vi "Make Defect Pair.vi"(4 "Maximum Distnce":dbl=12.0, 6 "Minimum Distance":dbl=11.0, 8 "Defect 2":cluster{"Species":string, "Defect Type":string}={"Species"="Te", "Defect Type"="Interstitial, Tetra, Unlike atoms"}, 9 "Defect 1":cluster{"Species":string, "Defect Type":string}={"Species"="Te", "Defect Type"="Substitutional"}, 10 "Defect 1 Atom Index":i32=10, 11 "Input Structure":T1={"Structure Name"="Gamma8_64atom", "Lattice vector a"=[13.21796569573, 0.0, 0.0], "Lattice vector b"=[0.0, 13.21796569573, 0.0], "Lattice vector c"=[0.0, 0.0, 13.21796569573], "Atoms Array"=[{"Atom Name"="Cd", "Positions (Direct)"=[[0.0, 0.0, 0.0], [0.0, 0.0, 0.5], [0.0, 0.5, 0.0], [0.0, 0.5, 0.5], [0.5, 0.0, 0.0], [0.5, 0.0, 0.5], [0.5, 0.5, 0.0], [0.5, 0.5, 0.5], [0.0, 0.25, 0.25], [0.0, 0.25, 0.75], [0.0, 0.75, 0.25], [0.0, 0.75, 0.75], [0.5, 0.25, 0.25], [0.5, 0.25, 0.75], [0.5, 0.75, 0.25], [0.5, 0.75, 0.75], [0.25, 0.0, 0.25], [0.25, 0.0, 0.75], [0.25, 0.5, 0.25], [0.25, 0.5, 0.75], [0.75, 0.0, 0.25], [0.75, 0.0, 0.75], [0.75, 0.5, 0.25], [0.75, 0.5, 0.75], [0.25, 0.25, 0.0], [0.25, 0.25, 0.5], [0.25, 0.75, 0.0], [0.25, 0.75, 0.5], [0.75, 0.25, 0.0], [0.75, 0.25, 0.5], [0.75, 0.75, 0.0], [0.75, 0.75, 0.5]], "Positions (Cartesian)"=[[0.0, 0.0, 0.0], [0.0, 0.0, 6.608982847865], [0.0, 6.608982847865, 0.0], [0.0, 6.608982847865, 6.608982847865], [6.608982847865, 0.0, 0.0], [6.608982847865, 0.0, 6.608982847865], [6.608982847865, 6.608982847865, 0.0], [6.608982847865, 6.608982847865, 6.608982847865], [0.0, 3.3044914239325, 3.3044914239325], [0.0, 3.3044914239325, 9.913474271797499], [0.0, 9.913474271797499, 3.3044914239325], [0.0, 9.913474271797499, 9.913474271797499], [6.608982847865, 3.3044914239325, 3.3044914239325], [6.608982847865, 3.3044914239325, 9.913474271797499], [6.608982847865, 9.913474271797499, 3.3044914239325], [6.608982847865, 9.913474271797499, 9.913474271797499], [3.3044914239325, 0.0, 3.3044914239325], [3.3044914239325, 0.0, 9.913474271797499], [3.3044914239325, 6.608982847865, 3.3044914239325], [3.3044914239325, 6.608982847865, 9.913474271797499], [9.913474271797499, 0.0, 3.3044914239325], [9.913474271797499, 0.0, 9.913474271797499], [9.913474271797499, 6.608982847865, 3.3044914239325], [9.913474271797499, 6.608982847865, 9.913474271797499], [3.3044914239325, 3.3044914239325, 0.0], [3.3044914239325, 3.3044914239325, 6.608982847865], [3.3044914239325, 9.913474271797499, 0.0], [3.3044914239325, 9.913474271797499, 6.608982847865], [9.913474271797499, 3.3044914239325, 0.0], [9.913474271797499, 3.3044914239325, 6.608982847865], [9.913474271797499, 9.913474271797499, 0.0], [9.913474271797499, 9.913474271797499, 6.608982847865]]}, {"Atom Name"="Te", "Positions (Direct)"=[[0.125, 0.125, 0.125], [0.125, 0.125, 0.625], [0.125, 0.625, 0.125], [0.125, 0.625, 0.625], [0.625, 0.125, 0.125], [0.625, 0.125, 0.625], [0.625, 0.625, 0.125], [0.625, 0.625, 0.625], [0.375, 0.375, 0.125], [0.375, 0.375, 0.625], [0.375, 0.875, 0.125], [0.375, 0.875, 0.625], [0.875, 0.375, 0.125], [0.875, 0.375, 0.625], [0.875, 0.875, 0.125], [0.875, 0.875, 0.625], [0.375, 0.125, 0.375], [0.375, 0.125, 0.875], [0.375, 0.625, 0.375], [0.375, 0.625, 0.875], [0.875, 0.125, 0.375], [0.875, 0.125, 0.875], [0.875, 0.625, 0.375], [0.875, 0.625, 0.875], [0.125, 0.375, 0.375], [0.125, 0.375, 0.875], [0.125, 0.875, 0.375], [0.125, 0.875, 0.875], [0.625, 0.375, 0.375], [0.625, 0.375, 0.875], [0.625, 0.875, 0.375], [0.625, 0.875, 0.875]], "Positions (Cartesian)"=[[1.65224571196625, 1.65224571196625, 1.65224571196625], [1.65224571196625, 1.65224571196625, 8.261228559831249], [1.65224571196625, 8.261228559831249, 1.65224571196625], [1.65224571196625, 8.261228559831249, 8.261228559831249], [8.261228559831249, 1.65224571196625, 1.65224571196625], [8.261228559831249, 1.65224571196625, 8.261228559831249], [8.261228559831249, 8.261228559831249, 1.65224571196625], [8.261228559831249, 8.261228559831249, 8.261228559831249], [4.9567371358987495, 4.9567371358987495, 1.65224571196625], [4.9567371358987495, 4.9567371358987495, 8.261228559831249], [4.9567371358987495, 11.56571998376375, 1.65224571196625], [4.9567371358987495, 11.56571998376375, 8.261228559831249], [11.56571998376375, 4.9567371358987495, 1.65224571196625], [11.56571998376375, 4.9567371358987495, 8.261228559831249], [11.56571998376375, 11.56571998376375, 1.65224571196625], [11.56571998376375, 11.56571998376375, 8.261228559831249], [4.9567371358987495, 1.65224571196625, 4.9567371358987495], [4.9567371358987495, 1.65224571196625, 11.56571998376375], [4.9567371358987495, 8.261228559831249, 4.9567371358987495], [4.9567371358987495, 8.261228559831249, 11.56571998376375], [11.56571998376375, 1.65224571196625, 4.9567371358987495], [11.56571998376375, 1.65224571196625, 11.56571998376375], [11.56571998376375, 8.261228559831249, 4.9567371358987495], [11.56571998376375, 8.261228559831249, 11.56571998376375], [1.65224571196625, 4.9567371358987495, 4.9567371358987495], [1.65224571196625, 4.9567371358987495, 11.56571998376375], [1.65224571196625, 11.56571998376375, 4.9567371358987495], [1.65224571196625, 11.56571998376375, 11.56571998376375], [8.261228559831249, 4.9567371358987495, 4.9567371358987495], [8.261228559831249, 4.9567371358987495, 11.56571998376375], [8.261228559831249, 11.56571998376375, 4.9567371358987495], [8.261228559831249, 11.56571998376375, 11.56571998376375]]}], "# of atoms"=64}) -> (0 "MATCH FOUND?!":bool=TRUE, 1 "Distance between defects (A)":dbl=11.799394498373799, 2 "Defect Options":T2(array[cluster])=[{"Distance from 1"=6.608982847864999, "Index"=32, "Position (Direct)"=[0.0, 0.25, 0.25], "Position (Cartesian)"=[0.0, 3.3044914239325, 3.3044914239325]}, {"Distance from 1"=6.608982847864999, "Index"=40, "Position (Direct)"=[0.0, 0.75, 0.75], "Position (Cartesian)"=[0.0, 9.913474271797499, 9.913474271797499]}, {"Distance from 1"=6.608982847864999, "Index"=46, "Position (Direct)"=[0.0, 1.25, 0.25], "Position (Cartesian)"=[0.0, 16.522457119662498, 3.3044914239325]}, {"Distance from 1"=6.608982847865, "Index"=88, "Position (Direct)"=[0.5, 0.75, 0.25], "Position (Cartesian)"=[6.608982847865, 9.913474271797499, 3.3044914239325]}, {"Distance from 1"=6.608982847865001, "Index"=38, "Position (Direct)"=[0.0, 0.75, -0.25000000000000006], "Position (Cartesian)"=[0.0, 9.913474271797499, -3.3044914239325003]}, {"Distance from 1"=8.094317848037637, "Index"=7, "Position (Direct)"=[-0.25000000000000006, 0.25, 0.0], "Position (Cartesian)"=[-3.3044914239325003, 3.3044914239325, 0.0]}, {"Distance from 1"=8.094317848037637, "Index"=8, "Position (Direct)"=[-0.25000000000000006, 0.25, 0.5], "Position (Cartesian)"=[-3.3044914239325003, 3.3044914239325, 6.608982847865]}, {"Distance from 1"=8.094317848037637, "Index"=12, "Position (Direct)"=[-0.25000000000000006, 0.5, 0.75], "Position (Cartesian)"=[-3.3044914239325003, 6.608982847865, 9.913474271797499]}, {"Distance from 1"=8.094317848037637, "Index"=19, "Position (Direct)"=[-0.25000000000000006, 1.0, 0.75], "Position (Cartesian)"=[-3.3044914239325003, 13.21796569573, 9.913474271797499]}, {"Distance from 1"=8.094317848037637, "Index"=21, "Position (Direct)"=[-0.25000000000000006, 1.25, 0.0], "Position (Cartesian)"=[-3.3044914239325003, 16.522457119662498, 0.0]}, {"Distance from 1"=8.094317848037637, "Index"=22, "Position (Direct)"=[-0.25000000000000006, 1.25, 0.5], "Position (Cartesian)"=[-3.3044914239325003, 16.522457119662498, 6.608982847865]}, {"Distance from 1"=8.094317848037637, "Index"=56, "Position (Direct)"=[0.25, 0.25, 0.0], "Position (Cartesian)"=[3.3044914239325, 3.3044914239325, 0.0]}, {"Distance from 1"=8.094317848037637, "Index"=57, "Position (Direct)"=[0.25, 0.25, 0.5], "Position (Cartesian)"=[3.3044914239325, 3.3044914239325, 6.608982847865]}, {"Distance from 1"=8.094317848037637, "Index"=59, "Position (Direct)"=[0.25, 0.5, -0.25000000000000006], "Position (Cartesian)"=[3.3044914239325, 6.608982847865, -3.3044914239325003]}, {"Distance from 1"=8.094317848037637, "Index"=61, "Position (Direct)"=[0.25, 0.5, 0.75], "Position (Cartesian)"=[3.3044914239325, 6.608982847865, 9.913474271797499]}, {"Distance from 1"=8.094317848037637, "Index"=68, "Position (Direct)"=[0.25, 1.0, 0.75], "Position (Cartesian)"=[3.3044914239325, 13.21796569573, 9.913474271797499]}, {"Distance from 1"=8.094317848037637, "Index"=70, "Position (Direct)"=[0.25, 1.25, 0.0], "Position (Cartesian)"=[3.3044914239325, 16.522457119662498, 0.0]}, {"Distance from 1"=8.094317848037637, "Index"=71, "Position (Direct)"=[0.25, 1.25, 0.5], "Position (Cartesian)"=[3.3044914239325, 16.522457119662498, 6.608982847865]}, {"Distance from 1"=8.094317848037637, "Index"=84, "Position (Direct)"=[0.5, 0.5, 0.0], "Position (Cartesian)"=[6.608982847865, 6.608982847865, 0.0]}, {"Distance from 1"=8.094317848037637, "Index"=85, "Position (Direct)"=[0.5, 0.5, 0.5], "Position (Cartesian)"=[6.608982847865, 6.608982847865, 6.608982847865]}, {"Distance from 1"=8.094317848037637, "Index"=91, "Position (Direct)"=[0.5, 1.0, 0.0], "Position (Cartesian)"=[6.608982847865, 13.21796569573, 0.0]}, {"Distance from 1"=8.094317848037637, "Index"=92, "Position (Direct)"=[0.5, 1.0, 0.5], "Position (Cartesian)"=[6.608982847865, 13.21796569573, 6.608982847865]}, {"Distance from 1"=8.094317848037639, "Index"=10, "Position (Direct)"=[-0.25000000000000006, 0.5, -0.25000000000000006], "Position (Cartesian)"=[-3.3044914239325003, 6.608982847865, -3.3044914239325003]}, {"Distance from 1"=8.094317848037639, "Index"=17, "Position (Direct)"=[-0.25000000000000006, 1.0, -0.25000000000000006], "Position (Cartesian)"=[-3.3044914239325003, 13.21796569573, -3.3044914239325003]}, {"Distance from 1"=8.094317848037639, "Index"=66, "Position (Direct)"=[0.25, 1.0, -0.25000000000000006], "Position (Cartesian)"=[3.3044914239325, 13.21796569573, -3.3044914239325003]}, {"Distance from 1"=9.346513176941842, "Index"=33, "Position (Direct)"=[0.0, 0.25, 0.75], "Position (Cartesian)"=[0.0, 3.3044914239325, 9.913474271797499]}, {"Distance from 1"=9.346513176941842, "Index"=47, "Position (Direct)"=[0.0, 1.25, 0.75], "Position (Cartesian)"=[0.0, 16.522457119662498, 9.913474271797499]}, {"Distance from 1"=9.346513176941844, "Index"=31, "Position (Direct)"=[0.0, 0.25, -0.25000000000000006], "Position (Cartesian)"=[0.0, 3.3044914239325, -3.3044914239325003]}, {"Distance from 1"=9.346513176941844, "Index"=45, "Position (Direct)"=[0.0, 1.25, -0.25000000000000006], "Position (Cartesian)"=[0.0, 16.522457119662498, -3.3044914239325003]}, {"Distance from 1"=9.346513176941844, "Index"=81, "Position (Direct)"=[0.5, 0.25, 0.25], "Position (Cartesian)"=[6.608982847865, 3.3044914239325, 3.3044914239325]}, {"Distance from 1"=9.346513176941844, "Index"=87, "Position (Direct)"=[0.5, 0.75, -0.25000000000000006], "Position (Cartesian)"=[6.608982847865, 9.913474271797499, -3.3044914239325003]}, {"Distance from 1"=9.346513176941844, "Index"=89, "Position (Direct)"=[0.5, 0.75, 0.75], "Position (Cartesian)"=[6.608982847865, 9.913474271797499, 9.913474271797499]}, {"Distance from 1"=9.346513176941844, "Index"=95, "Position (Direct)"=[0.5, 1.25, 0.25], "Position (Cartesian)"=[6.608982847865, 16.522457119662498, 3.3044914239325]}, {"Distance from 1"=10.44971940811974, "Index"=4, "Position (Direct)"=[-0.25000000000000006, 0.0, 0.25], "Position (Cartesian)"=[-3.3044914239325003, 0.0, 3.3044914239325]}, {"Distance from 1"=10.44971940811974, "Index"=16, "Position (Direct)"=[-0.25000000000000006, 0.75, 1.0], "Position (Cartesian)"=[-3.3044914239325003, 9.913474271797499, 13.21796569573]}, {"Distance from 1"=10.44971940811974, "Index"=28, "Position (Direct)"=[0.0, 0.0, 0.0], "Position (Cartesian)"=[0.0, 0.0, 0.0]}, {"Distance from 1"=10.44971940811974, "Index"=29, "Position (Direct)"=[0.0, 0.0, 0.5], "Position (Cartesian)"=[0.0, 0.0, 6.608982847865]}, {"Distance from 1"=10.44971940811974, "Index"=37, "Position (Direct)"=[0.0, 0.5, 1.0], "Position (Cartesian)"=[0.0, 6.608982847865, 13.21796569573]}, {"Distance from 1"=10.44971940811974, "Index"=44, "Position (Direct)"=[0.0, 1.0, 1.0], "Position (Cartesian)"=[0.0, 13.21796569573, 13.21796569573]}, {"Distance from 1"=10.44971940811974, "Index"=53, "Position (Direct)"=[0.25, 0.0, 0.25], "Position (Cartesian)"=[3.3044914239325, 0.0, 3.3044914239325]}, {"Distance from 1"=10.44971940811974, "Index"=65, "Position (Direct)"=[0.25, 0.75, 1.0], "Position (Cartesian)"=[3.3044914239325, 9.913474271797499, 13.21796569573]}, {"Distance from 1"=10.44971940811974, "Index"=109, "Position (Direct)"=[0.75, 0.5, 0.25], "Position (Cartesian)"=[9.913474271797499, 6.608982847865, 3.3044914239325]}, {"Distance from 1"=10.44971940811974, "Index"=112, "Position (Direct)"=[0.75, 0.75, 0.0], "Position (Cartesian)"=[9.913474271797499, 9.913474271797499, 0.0]}, {"Distance from 1"=10.44971940811974, "Index"=113, "Position (Direct)"=[0.75, 0.75, 0.5], "Position (Cartesian)"=[9.913474271797499, 9.913474271797499, 6.608982847865]}, {"Distance from 1"=10.44971940811974, "Index"=116, "Position (Direct)"=[0.75, 1.0, 0.25], "Position (Cartesian)"=[9.913474271797499, 13.21796569573, 3.3044914239325]}, {"Distance from 1"=11.44709407885343, "Index"=80, "Position (Direct)"=[0.5, 0.25, -0.25000000000000006], "Position (Cartesian)"=[6.608982847865, 3.3044914239325, -3.3044914239325003]}, {"Distance from 1"=11.44709407885343, "Index"=82, "Position (Direct)"=[0.5, 0.25, 0.75], "Position (Cartesian)"=[6.608982847865, 3.3044914239325, 9.913474271797499]}, {"Distance from 1"=11.44709407885343, "Index"=94, "Position (Direct)"=[0.5, 1.25, -0.25000000000000006], "Position (Cartesian)"=[6.608982847865, 16.522457119662498, -3.3044914239325003]}, {"Distance from 1"=11.44709407885343, "Index"=96, "Position (Direct)"=[0.5, 1.25, 0.75], "Position (Cartesian)"=[6.608982847865, 16.522457119662498, 9.913474271797499]}, {"Distance from 1"=12.364274745888176, "Index"=110, "Position (Direct)"=[0.75, 0.5, 0.75], "Position (Cartesian)"=[9.913474271797499, 6.608982847865, 9.913474271797499]}, {"Distance from 1"=12.364274745888178, "Index"=3, "Position (Direct)"=[-0.25000000000000006, 0.0, -0.25000000000000006], "Position (Cartesian)"=[-3.3044914239325003, 0.0, -3.3044914239325003]}, {"Distance from 1"=12.364274745888178, "Index"=5, "Position (Direct)"=[-0.25000000000000006, 0.0, 0.75], "Position (Cartesian)"=[-3.3044914239325003, 0.0, 9.913474271797499]}, {"Distance from 1"=12.364274745888178, "Index"=9, "Position (Direct)"=[-0.25000000000000006, 0.25, 1.0], "Position (Cartesian)"=[-3.3044914239325003, 3.3044914239325, 13.21796569573]}, {"Distance from 1"=12.364274745888178, "Index"=23, "Position (Direct)"=[-0.25000000000000006, 1.25, 1.0], "Position (Cartesian)"=[-3.3044914239325003, 16.522457119662498, 13.21796569573]}, {"Distance from 1"=12.364274745888178, "Index"=52, "Position (Direct)"=[0.25, 0.0, -0.25000000000000006], "Position (Cartesian)"=[3.3044914239325, 0.0, -3.3044914239325003]}, {"Distance from 1"=12.364274745888178, "Index"=54, "Position (Direct)"=[0.25, 0.0, 0.75], "Position (Cartesian)"=[3.3044914239325, 0.0, 9.913474271797499]}, {"Distance from 1"=12.364274745888178, "Index"=58, "Position (Direct)"=[0.25, 0.25, 1.0], "Position (Cartesian)"=[3.3044914239325, 3.3044914239325, 13.21796569573]}, {"Distance from 1"=12.364274745888178, "Index"=72, "Position (Direct)"=[0.25, 1.25, 1.0], "Position (Cartesian)"=[3.3044914239325, 16.522457119662498, 13.21796569573]}, {"Distance from 1"=12.364274745888178, "Index"=77, "Position (Direct)"=[0.5, 0.0, 0.0], "Position (Cartesian)"=[6.608982847865, 0.0, 0.0]}, {"Distance from 1"=12.364274745888178, "Index"=78, "Position (Direct)"=[0.5, 0.0, 0.5], "Position (Cartesian)"=[6.608982847865, 0.0, 6.608982847865]}, {"Distance from 1"=12.364274745888178, "Index"=86, "Position (Direct)"=[0.5, 0.5, 1.0], "Position (Cartesian)"=[6.608982847865, 6.608982847865, 13.21796569573]}, {"Distance from 1"=12.364274745888178, "Index"=93, "Position (Direct)"=[0.5, 1.0, 1.0], "Position (Cartesian)"=[6.608982847865, 13.21796569573, 13.21796569573]}, {"Distance from 1"=12.364274745888178, "Index"=105, "Position (Direct)"=[0.75, 0.25, 0.0], "Position (Cartesian)"=[9.913474271797499, 3.3044914239325, 0.0]}, {"Distance from 1"=12.364274745888178, "Index"=106, "Position (Direct)"=[0.75, 0.25, 0.5], "Position (Cartesian)"=[9.913474271797499, 3.3044914239325, 6.608982847865]}, {"Distance from 1"=12.364274745888178, "Index"=108, "Position (Direct)"=[0.75, 0.5, -0.25000000000000006], "Position (Cartesian)"=[9.913474271797499, 6.608982847865, -3.3044914239325003]}, {"Distance from 1"=12.364274745888178, "Index"=115, "Position (Direct)"=[0.75, 1.0, -0.25000000000000006], "Position (Cartesian)"=[9.913474271797499, 13.21796569573, -3.3044914239325003]}, {"Distance from 1"=12.364274745888178, "Index"=117, "Position (Direct)"=[0.75, 1.0, 0.75], "Position (Cartesian)"=[9.913474271797499, 13.21796569573, 9.913474271797499]}, {"Distance from 1"=12.364274745888178, "Index"=119, "Position (Direct)"=[0.75, 1.25, 0.0], "Position (Cartesian)"=[9.913474271797499, 16.522457119662498, 0.0]}, {"Distance from 1"=12.364274745888178, "Index"=120, "Position (Direct)"=[0.75, 1.25, 0.5], "Position (Cartesian)"=[9.913474271797499, 16.522457119662498, 6.608982847865]}, {"Distance from 1"=13.217965695729998, "Index"=41, "Position (Direct)"=[0.0, 0.75, 1.25], "Position (Cartesian)"=[0.0, 9.913474271797499, 16.522457119662498]}, {"Distance from 1"=13.21796569573, "Index"=25, "Position (Direct)"=[0.0, -0.25000000000000006, 0.25], "Position (Cartesian)"=[0.0, -3.3044914239325003, 3.3044914239325]}, {"Distance from 1"=13.21796569573, "Index"=137, "Position (Direct)"=[1.0, 0.75, 0.25], "Position (Cartesian)"=[13.21796569573, 9.913474271797499, 3.3044914239325]}, {"Distance from 1"=14.019769765412764, "Index"=13, "Position (Direct)"=[-0.25000000000000006, 0.5, 1.25], "Position (Cartesian)"=[-3.3044914239325003, 6.608982847865, 16.522457119662498]}, {"Distance from 1"=14.019769765412764, "Index"=20, "Position (Direct)"=[-0.25000000000000006, 1.0, 1.25], "Position (Cartesian)"=[-3.3044914239325003, 13.21796569573, 16.522457119662498]}, {"Distance from 1"=14.019769765412764, "Index"=62, "Position (Direct)"=[0.25, 0.5, 1.25], "Position (Cartesian)"=[3.3044914239325, 6.608982847865, 16.522457119662498]}, {"Distance from 1"=14.019769765412764, "Index"=69, "Position (Direct)"=[0.25, 1.0, 1.25], "Position (Cartesian)"=[3.3044914239325, 13.21796569573, 16.522457119662498]}, {"Distance from 1"=14.019769765412766, "Index"=0, "Position (Direct)"=[-0.25000000000000006, -0.25000000000000006, 0.0], "Position (Cartesian)"=[-3.3044914239325003, -3.3044914239325003, 0.0]}, {"Distance from 1"=14.019769765412766, "Index"=1, "Position (Direct)"=[-0.25000000000000006, -0.25000000000000006, 0.5], "Position (Cartesian)"=[-3.3044914239325003, -3.3044914239325003, 6.608982847865]}, {"Distance from 1"=14.019769765412766, "Index"=30, "Position (Direct)"=[0.0, 0.0, 1.0], "Position (Cartesian)"=[0.0, 0.0, 13.21796569573]}, {"Distance from 1"=14.019769765412766, "Index"=49, "Position (Direct)"=[0.25, -0.25000000000000006, 0.0], "Position (Cartesian)"=[3.3044914239325, -3.3044914239325003, 0.0]}, {"Distance from 1"=14.019769765412766, "Index"=50, "Position (Direct)"=[0.25, -0.25000000000000006, 0.5], "Position (Cartesian)"=[3.3044914239325, -3.3044914239325003, 6.608982847865]}, {"Distance from 1"=14.019769765412766, "Index"=102, "Position (Direct)"=[0.75, 0.0, 0.25], "Position (Cartesian)"=[9.913474271797499, 0.0, 3.3044914239325]}, {"Distance from 1"=14.019769765412766, "Index"=114, "Position (Direct)"=[0.75, 0.75, 1.0], "Position (Cartesian)"=[9.913474271797499, 9.913474271797499, 13.21796569573]}, {"Distance from 1"=14.019769765412766, "Index"=133, "Position (Direct)"=[1.0, 0.5, 0.0], "Position (Cartesian)"=[13.21796569573, 6.608982847865, 0.0]}, {"Distance from 1"=14.019769765412766, "Index"=134, "Position (Direct)"=[1.0, 0.5, 0.5], "Position (Cartesian)"=[13.21796569573, 6.608982847865, 6.608982847865]}, {"Distance from 1"=14.019769765412766, "Index"=140, "Position (Direct)"=[1.0, 1.0, 0.0], "Position (Cartesian)"=[13.21796569573, 13.21796569573, 0.0]}, {"Distance from 1"=14.019769765412766, "Index"=141, "Position (Direct)"=[1.0, 1.0, 0.5], "Position (Cartesian)"=[13.21796569573, 13.21796569573, 6.608982847865]}, {"Distance from 1"=14.778134909956288, "Index"=34, "Position (Direct)"=[0.0, 0.25, 1.25], "Position (Cartesian)"=[0.0, 3.3044914239325, 16.522457119662498]}, {"Distance from 1"=14.778134909956288, "Index"=48, "Position (Direct)"=[0.0, 1.25, 1.25], "Position (Cartesian)"=[0.0, 16.522457119662498, 16.522457119662498]}, {"Distance from 1"=14.778134909956288, "Index"=90, "Position (Direct)"=[0.5, 0.75, 1.25], "Position (Cartesian)"=[6.608982847865, 9.913474271797499, 16.522457119662498]}, {"Distance from 1"=14.77813490995629, "Index"=26, "Position (Direct)"=[0.0, -0.25000000000000006, 0.75], "Position (Cartesian)"=[0.0, -3.3044914239325003, 9.913474271797499]}, {"Distance from 1"=14.77813490995629, "Index"=74, "Position (Direct)"=[0.5, -0.25000000000000006, 0.25], "Position (Cartesian)"=[6.608982847865, -3.3044914239325003, 3.3044914239325]}, {"Distance from 1"=14.77813490995629, "Index"=130, "Position (Direct)"=[1.0, 0.25, 0.25], "Position (Cartesian)"=[13.21796569573, 3.3044914239325, 3.3044914239325]}, {"Distance from 1"=14.77813490995629, "Index"=138, "Position (Direct)"=[1.0, 0.75, 0.75], "Position (Cartesian)"=[13.21796569573, 9.913474271797499, 9.913474271797499]}, {"Distance from 1"=14.77813490995629, "Index"=144, "Position (Direct)"=[1.0, 1.25, 0.25], "Position (Cartesian)"=[13.21796569573, 16.522457119662498, 3.3044914239325]}, {"Distance from 1"=14.778134909956291, "Index"=24, "Position (Direct)"=[0.0, -0.25000000000000006, -0.25000000000000006], "Position (Cartesian)"=[0.0, -3.3044914239325003, -3.3044914239325003]}, {"Distance from 1"=14.778134909956291, "Index"=136, "Position (Direct)"=[1.0, 0.75, -0.25000000000000006], "Position (Cartesian)"=[13.21796569573, 9.913474271797499, -3.3044914239325003]}, {"Distance from 1"=15.499438653014362, "Index"=79, "Position (Direct)"=[0.5, 0.0, 1.0], "Position (Cartesian)"=[6.608982847865, 0.0, 13.21796569573]}, {"Distance from 1"=15.499438653014362, "Index"=101, "Position (Direct)"=[0.75, 0.0, -0.25000000000000006], "Position (Cartesian)"=[9.913474271797499, 0.0, -3.3044914239325003]}, {"Distance from 1"=15.499438653014362, "Index"=103, "Position (Direct)"=[0.75, 0.0, 0.75], "Position (Cartesian)"=[9.913474271797499, 0.0, 9.913474271797499]}, {"Distance from 1"=15.499438653014362, "Index"=107, "Position (Direct)"=[0.75, 0.25, 1.0], "Position (Cartesian)"=[9.913474271797499, 3.3044914239325, 13.21796569573]}, {"Distance from 1"=15.499438653014362, "Index"=121, "Position (Direct)"=[0.75, 1.25, 1.0], "Position (Cartesian)"=[9.913474271797499, 16.522457119662498, 13.21796569573]}, {"Distance from 1"=16.188635696075274, "Index"=73, "Position (Direct)"=[0.5, -0.25000000000000006, -0.25000000000000006], "Position (Cartesian)"=[6.608982847865, -3.3044914239325003, -3.3044914239325003]}, {"Distance from 1"=16.188635696075274, "Index"=75, "Position (Direct)"=[0.5, -0.25000000000000006, 0.75], "Position (Cartesian)"=[6.608982847865, -3.3044914239325003, 9.913474271797499]}, {"Distance from 1"=16.188635696075274, "Index"=83, "Position (Direct)"=[0.5, 0.25, 1.25], "Position (Cartesian)"=[6.608982847865, 3.3044914239325, 16.522457119662498]}, {"Distance from 1"=16.188635696075274, "Index"=97, "Position (Direct)"=[0.5, 1.25, 1.25], "Position (Cartesian)"=[6.608982847865, 16.522457119662498, 16.522457119662498]}, {"Distance from 1"=16.188635696075274, "Index"=129, "Position (Direct)"=[1.0, 0.25, -0.25000000000000006], "Position (Cartesian)"=[13.21796569573, 3.3044914239325, -3.3044914239325003]}, {"Distance from 1"=16.188635696075274, "Index"=131, "Position (Direct)"=[1.0, 0.25, 0.75], "Position (Cartesian)"=[13.21796569573, 3.3044914239325, 9.913474271797499]}, {"Distance from 1"=16.188635696075274, "Index"=143, "Position (Direct)"=[1.0, 1.25, -0.25000000000000006], "Position (Cartesian)"=[13.21796569573, 16.522457119662498, -3.3044914239325003]}, {"Distance from 1"=16.188635696075274, "Index"=145, "Position (Direct)"=[1.0, 1.25, 0.75], "Position (Cartesian)"=[13.21796569573, 16.522457119662498, 9.913474271797499]}, {"Distance from 1"=16.849666253131822, "Index"=6, "Position (Direct)"=[-0.25000000000000006, 0.0, 1.25], "Position (Cartesian)"=[-3.3044914239325003, 0.0, 16.522457119662498]}, {"Distance from 1"=16.849666253131822, "Index"=55, "Position (Direct)"=[0.25, 0.0, 1.25], "Position (Cartesian)"=[3.3044914239325, 0.0, 16.522457119662498]}, {"Distance from 1"=16.849666253131822, "Index"=111, "Position (Direct)"=[0.75, 0.5, 1.25], "Position (Cartesian)"=[9.913474271797499, 6.608982847865, 16.522457119662498]}, {"Distance from 1"=16.849666253131822, "Index"=118, "Position (Direct)"=[0.75, 1.0, 1.25], "Position (Cartesian)"=[9.913474271797499, 13.21796569573, 16.522457119662498]}, {"Distance from 1"=16.849666253131822, "Index"=135, "Position (Direct)"=[1.0, 0.5, 1.0], "Position (Cartesian)"=[13.21796569573, 6.608982847865, 13.21796569573]}, {"Distance from 1"=16.849666253131822, "Index"=158, "Position (Direct)"=[1.25, 0.5, 0.25], "Position (Cartesian)"=[16.522457119662498, 6.608982847865, 3.3044914239325]}, {"Distance from 1"=16.849666253131822, "Index"=161, "Position (Direct)"=[1.25, 0.75, 0.0], "Position (Cartesian)"=[16.522457119662498, 9.913474271797499, 0.0]}, {"Distance from 1"=16.849666253131822, "Index"=162, "Position (Direct)"=[1.25, 0.75, 0.5], "Position (Cartesian)"=[16.522457119662498, 9.913474271797499, 6.608982847865]}, {"Distance from 1"=16.849666253131822, "Index"=165, "Position (Direct)"=[1.25, 1.0, 0.25], "Position (Cartesian)"=[16.522457119662498, 13.21796569573, 3.3044914239325]}, {"Distance from 1"=16.849666253131826, "Index"=2, "Position (Direct)"=[-0.25000000000000006, -0.25000000000000006, 1.0], "Position (Cartesian)"=[-3.3044914239325003, -3.3044914239325003, 13.21796569573]}, {"Distance from 1"=16.849666253131826, "Index"=51, "Position (Direct)"=[0.25, -0.25000000000000006, 1.0], "Position (Cartesian)"=[3.3044914239325, -3.3044914239325003, 13.21796569573]}, {"Distance from 1"=16.849666253131826, "Index"=98, "Position (Direct)"=[0.75, -0.25000000000000006, 0.0], "Position (Cartesian)"=[9.913474271797499, -3.3044914239325003, 0.0]}, {"Distance from 1"=16.849666253131826, "Index"=99, "Position (Direct)"=[0.75, -0.25000000000000006, 0.5], "Position (Cartesian)"=[9.913474271797499, -3.3044914239325003, 6.608982847865]}, {"Distance from 1"=16.849666253131826, "Index"=126, "Position (Direct)"=[1.0, 0.0, 0.0], "Position (Cartesian)"=[13.21796569573, 0.0, 0.0]}, {"Distance from 1"=16.849666253131826, "Index"=127, "Position (Direct)"=[1.0, 0.0, 0.5], "Position (Cartesian)"=[13.21796569573, 0.0, 6.608982847865]}, {"Distance from 1"=16.849666253131826, "Index"=142, "Position (Direct)"=[1.0, 1.0, 1.0], "Position (Cartesian)"=[13.21796569573, 13.21796569573, 13.21796569573]}], 3 "Defectuous Structure":T1={"Structure Name"="Gamma8_64atom", "Lattice vector a"=[13.21796569573, 0.0, 0.0], "Lattice vector b"=[0.0, 13.21796569573, 0.0], "Lattice vector c"=[0.0, 0.0, 13.21796569573], "Atoms Array"=[{"Atom Name"="Cd", "Positions (Direct)"=[[0.0, 0.0, 0.0], [0.0, 0.0, 0.5], [0.0, 0.5, 0.0], [0.0, 0.5, 0.5], [0.5, 0.0, 0.0], [0.5, 0.0, 0.5], [0.5, 0.5, 0.0], [0.5, 0.5, 0.5], [0.0, 0.25, 0.25], [0.0, 0.25, 0.75], [0.0, 0.75, 0.75], [0.5, 0.25, 0.25], [0.5, 0.25, 0.75], [0.5, 0.75, 0.25], [0.5, 0.75, 0.75], [0.25, 0.0, 0.25], [0.25, 0.0, 0.75], [0.25, 0.5, 0.25], [0.25, 0.5, 0.75], [0.75, 0.0, 0.25], [0.75, 0.0, 0.75], [0.75, 0.5, 0.25], [0.75, 0.5, 0.75], [0.25, 0.25, 0.0], [0.25, 0.25, 0.5], [0.25, 0.75, 0.0], [0.25, 0.75, 0.5], [0.75, 0.25, 0.0], [0.75, 0.25, 0.5], [0.75, 0.75, 0.0], [0.75, 0.75, 0.5]], "Positions (Cartesian)"=[[0.0, 0.0, 0.0], [0.0, 0.0, 6.608982847865], [0.0, 6.608982847865, 0.0], [0.0, 6.608982847865, 6.608982847865], [6.608982847865, 0.0, 0.0], [6.608982847865, 0.0, 6.608982847865], [6.608982847865, 6.608982847865, 0.0], [6.608982847865, 6.608982847865, 6.608982847865], [0.0, 3.3044914239325, 3.3044914239325], [0.0, 3.3044914239325, 9.913474271797499], [0.0, 9.913474271797499, 9.913474271797499], [6.608982847865, 3.3044914239325, 3.3044914239325], [6.608982847865, 3.3044914239325, 9.913474271797499], [6.608982847865, 9.913474271797499, 3.3044914239325], [6.608982847865, 9.913474271797499, 9.913474271797499], [3.3044914239325, 0.0, 3.3044914239325], [3.3044914239325, 0.0, 9.913474271797499], [3.3044914239325, 6.608982847865, 3.3044914239325], [3.3044914239325, 6.608982847865, 9.913474271797499], [9.913474271797499, 0.0, 3.3044914239325], [9.913474271797499, 0.0, 9.913474271797499], [9.913474271797499, 6.608982847865, 3.3044914239325], [9.913474271797499, 6.608982847865, 9.913474271797499], [3.3044914239325, 3.3044914239325, 0.0], [3.3044914239325, 3.3044914239325, 6.608982847865], [3.3044914239325, 9.913474271797499, 0.0], [3.3044914239325, 9.913474271797499, 6.608982847865], [9.913474271797499, 3.3044914239325, 0.0], [9.913474271797499, 3.3044914239325, 6.608982847865], [9.913474271797499, 9.913474271797499, 0.0], [9.913474271797499, 9.913474271797499, 6.608982847865]]}, {"Atom Name"="Te", "Positions (Direct)"=[[0.125, 0.125, 0.125], [0.125, 0.125, 0.625], [0.125, 0.625, 0.125], [0.125, 0.625, 0.625], [0.625, 0.125, 0.125], [0.625, 0.125, 0.625], [0.625, 0.625, 0.125], [0.625, 0.625, 0.625], [0.375, 0.375, 0.125], [0.375, 0.375, 0.625], [0.375, 0.875, 0.125], [0.375, 0.875, 0.625], [0.875, 0.375, 0.125], [0.875, 0.375, 0.625], [0.875, 0.875, 0.125], [0.875, 0.875, 0.625], [0.375, 0.125, 0.375], [0.375, 0.125, 0.875], [0.375, 0.625, 0.375], [0.375, 0.625, 0.875], [0.875, 0.125, 0.375], [0.875, 0.125, 0.875], [0.875, 0.625, 0.375], [0.875, 0.625, 0.875], [0.125, 0.375, 0.375], [0.125, 0.375, 0.875], [0.125, 0.875, 0.375], [0.125, 0.875, 0.875], [0.625, 0.375, 0.375], [0.625, 0.375, 0.875], [0.625, 0.875, 0.375], [0.625, 0.875, 0.875], [0.0, 0.75, 0.25], [0.875, 0.625, 0.125]], "Positions (Cartesian)"=[[1.65224571196625, 1.65224571196625, 1.65224571196625], [1.65224571196625, 1.65224571196625, 8.261228559831249], [1.65224571196625, 8.261228559831249, 1.65224571196625], [1.65224571196625, 8.261228559831249, 8.261228559831249], [8.261228559831249, 1.65224571196625, 1.65224571196625], [8.261228559831249, 1.65224571196625, 8.261228559831249], [8.261228559831249, 8.261228559831249, 1.65224571196625], [8.261228559831249, 8.261228559831249, 8.261228559831249], [4.9567371358987495, 4.9567371358987495, 1.65224571196625], [4.9567371358987495, 4.9567371358987495, 8.261228559831249], [4.9567371358987495, 11.56571998376375, 1.65224571196625], [4.9567371358987495, 11.56571998376375, 8.261228559831249], [11.56571998376375, 4.9567371358987495, 1.65224571196625], [11.56571998376375, 4.9567371358987495, 8.261228559831249], [11.56571998376375, 11.56571998376375, 1.65224571196625], [11.56571998376375, 11.56571998376375, 8.261228559831249], [4.9567371358987495, 1.65224571196625, 4.9567371358987495], [4.9567371358987495, 1.65224571196625, 11.56571998376375], [4.9567371358987495, 8.261228559831249, 4.9567371358987495], [4.9567371358987495, 8.261228559831249, 11.56571998376375], [11.56571998376375, 1.65224571196625, 4.9567371358987495], [11.56571998376375, 1.65224571196625, 11.56571998376375], [11.56571998376375, 8.261228559831249, 4.9567371358987495], [11.56571998376375, 8.261228559831249, 11.56571998376375], [1.65224571196625, 4.9567371358987495, 4.9567371358987495], [1.65224571196625, 4.9567371358987495, 11.56571998376375], [1.65224571196625, 11.56571998376375, 4.9567371358987495], [1.65224571196625, 11.56571998376375, 11.56571998376375], [8.261228559831249, 4.9567371358987495, 4.9567371358987495], [8.261228559831249, 4.9567371358987495, 11.56571998376375], [8.261228559831249, 11.56571998376375, 4.9567371358987495], [8.261228559831249, 11.56571998376375, 11.56571998376375], [0.0, 9.913474271797499, 3.3044914239325], [11.56571998376375, 8.261228559831249, 1.65224571196625]]}], "# of atoms"=65})   [LabVIEW 2010]
uses:
  <vilib>/Analysis/_algsub.llb/Real Vector Norm.vi
  <vilib>/Analysis/NI_AALPro.lvlib
panel:
  out "Array":dbl[](array[numeric])=[0.0, 4.673256588470922, 4.673256588470922, 4.673256588470922, 4.673256588470922, 4.673256588470922, 4.673256588470922, 4.673256588470922, 4.673256588470922, 4.673256588470922, 4.673256588470922, 4.673256588470922, 4.673256588470923, 6.608982847864999, 6.608982847864999, 6.608982847864999, 6.608982847865, 6.608982847865001, 8.094317848037637, 8.094317848037637, 8.094317848037637, 8.094317848037637, 8.094317848037637, 8.094317848037637, 8.094317848037637, 8.094317848037637, 8.094317848037637, 8.094317848037637, 8.094317848037637, 8.094317848037637, 8.094317848037637, 8.094317848037637, 8.094317848037637, 8.094317848037637, 8.094317848037637, 8.094317848037639, 8.094317848037639, 8.094317848037639, 9.346513176941842, 9.346513176941842, 9.346513176941844, 9.346513176941844, 9.346513176941844, 9.346513176941844, 9.346513176941844, 9.346513176941844, 10.44971940811974, 10.44971940811974, 10.44971940811974, 10.44971940811974, 10.44971940811974, 10.44971940811974, 10.44971940811974, 10.44971940811974, 10.44971940811974, 10.44971940811974, 10.44971940811974, 10.44971940811974, 11.44709407885343, 11.44709407885343, 11.44709407885343, 11.44709407885343, 12.364274745888176, 12.364274745888178, 12.364274745888178, 12.364274745888178, 12.364274745888178, 12.364274745888178, 12.364274745888178, 12.364274745888178, 12.364274745888178, 12.364274745888178, 12.364274745888178, 12.364274745888178, 12.364274745888178, 12.364274745888178, 12.364274745888178, 12.364274745888178, 12.364274745888178, 12.364274745888178, 12.364274745888178, 12.364274745888178, 13.217965695729998, 13.21796569573, 13.21796569573, 14.019769765412764, 14.019769765412764, 14.019769765412764, 14.019769765412764, 14.019769765412766, 14.019769765412766, 14.019769765412766, 14.019769765412766, 14.019769765412766, 14.019769765412766, 14.019769765412766, 14.019769765412766, 14.019769765412766, 14.019769765412766, 14.019769765412766, 14.778134909956288, 14.778134909956288, 14.778134909956288, 14.77813490995629, 14.77813490995629, 14.77813490995629, 14.77813490995629, 14.77813490995629, 14.778134909956291, 14.778134909956291, 15.499438653014362, 15.499438653014362, 15.499438653014362, 15.499438653014362, 15.499438653014362, 16.188635696075274, 16.188635696075274, 16.188635696075274, 16.188635696075274, 16.188635696075274, 16.188635696075274, 16.188635696075274, 16.188635696075274, 16.849666253131822, 16.849666253131822, 16.849666253131822, 16.849666253131822, 16.849666253131822, 16.849666253131822, 16.849666253131822, 16.849666253131822, 16.849666253131822, 16.849666253131826, 16.849666253131826, 16.849666253131826, 16.849666253131826, 16.849666253131826, 16.849666253131826, 16.849666253131826, 18.099444939701968, 18.099444939701968, 18.099444939701968, 18.099444939701968, 18.099444939701968, 18.099444939701968, 18.099444939701968, 18.099444939701968, 18.69302635388369, 18.69302635388369, 18.69302635388369, 19.268330529879254, 19.268330529879254, 19.268330529879254, 19.268330529879254, 19.268330529879254, 19.826948543594998, 19.826948543594998, 19.826948543594998, 19.826948543594998, 19.826948543594998, 20.370253206380394, 20.370253206380394, 20.370253206380394, 20.370253206380394, 21.41555205861909, 21.41555205861909, 21.41555205861909, 21.41555205861909, 22.89418815770686, 23.36628294235461, 23.36628294235461]
  in  "Distance to check":dbl=6.0
  out "Numeric":i32
  out "Defect 2 (Cart)":dbl[](array[numeric])=[-1.6522457119662501, 8.261228559831249, 14.87021140769625]
  out "Defect 1 (Cart)":dbl[](array[numeric])=[0.0, 9.913474271797499, 3.3044914239325]
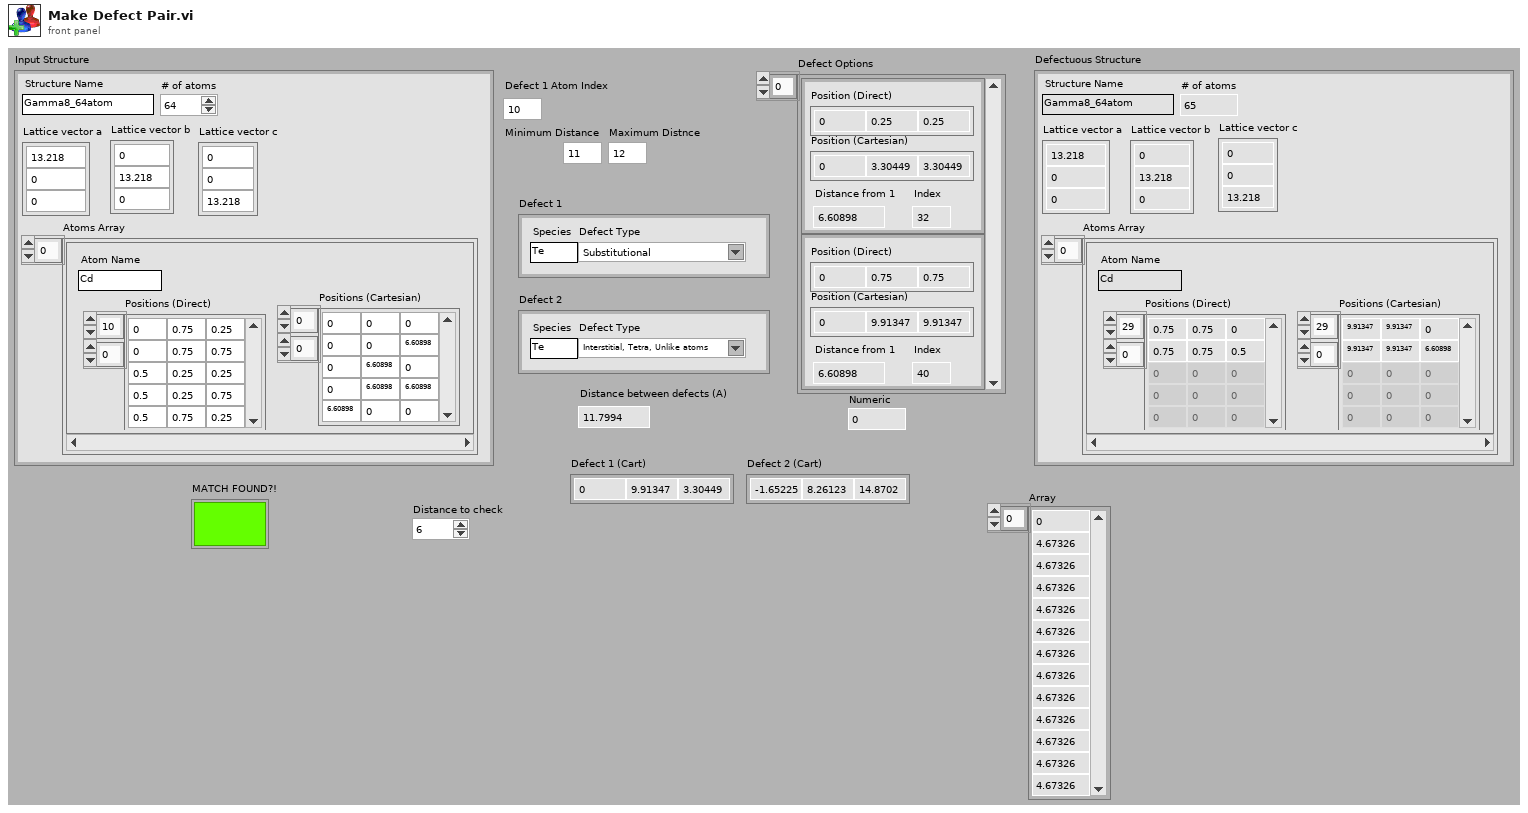
[diagram p1: front panel]
types:
  T1 = cluster{"Structure Name":string, "Lattice vector a":dbl[], "Lattice vector b":dbl[], "Lattice vector c":dbl[], "Atoms Array":cluster{"Atom Name":string, "Positions (Direct)":dbl[][], "Positions (Cartesian)":dbl[][]}[], "# of atoms":i32}
  T2 = cluster{"Distance from 1":dbl, "Index":i32, "Position (Direct)":dbl[], "Position (Cartesian)":dbl[]}[]
  T3 = cluster{"norm":dbl, i32, "Positions (Direct)":dbl[], "Positions (Cartesian)":dbl[]}[]
  T4 = cluster{"Atom Name":string, "Positions (Direct)":dbl[][], "Positions (Cartesian)":dbl[][]}[]
  T5 = cluster{"Atom Name":string, "Positions (Direct)":dbl[][], "Positions (Cartesian)":dbl[][]}
  T6 = enum16{"Tetrahedral (4 atoms)", "Octahedral (6 atoms)"}
  T7 = cluster{"norm":dbl, i32, "Positions (Direct)":dbl[], "Positions (Cartesian)":dbl[]}
  T8 = cluster{i32, "Positions (Direct)":dbl[], "Positions (Cartesian)":dbl[]}
  T9 = cluster{i32, "Positions (Direct)":dbl[], "Actual Position":dbl[]}
  T10 = cluster{"norm":dbl, i32, "Positions (Direct)":dbl[], "Actual Position":dbl[]}
  T11 = cluster{"Structure ID":string, "Lattice vector a":dbl[], "Lattice vector b":dbl[], "Lattice vector c":dbl[], "Atoms Array":cluster{"Atom Name":string, "Positions (Direct)":dbl[][], "Positions (Cartesian)":dbl[][]}[], "# of atoms":i32}
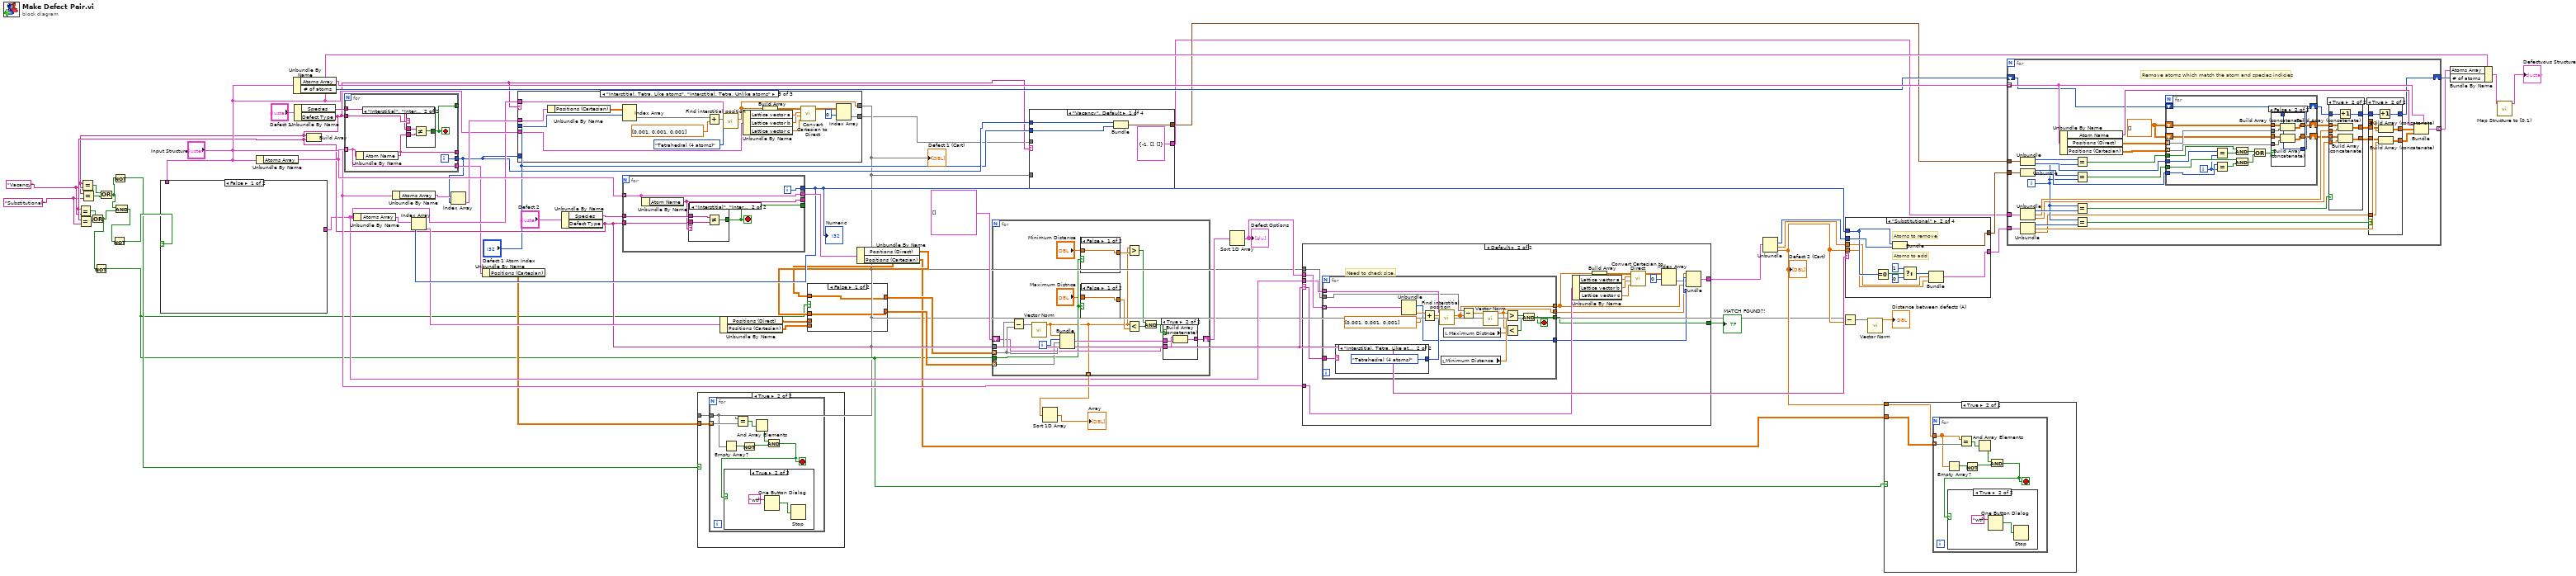
[diagram p0: block diagram]
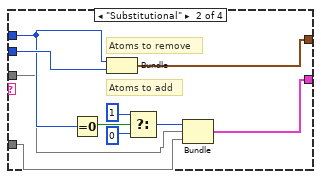
[diagram p2: hidden frame]
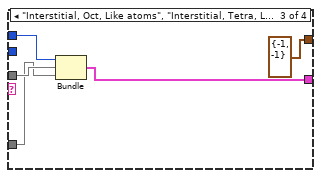
[diagram p3: hidden frame]
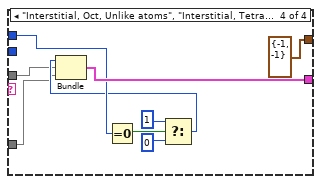
[diagram p4: hidden frame]
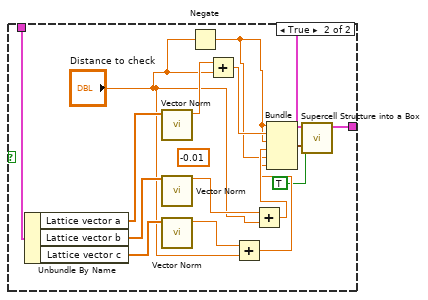
[diagram p10: hidden frame]
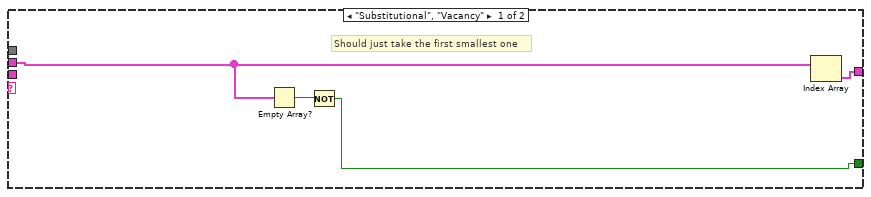
[diagram p11: hidden frame]
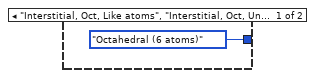
[diagram p12: hidden frame]
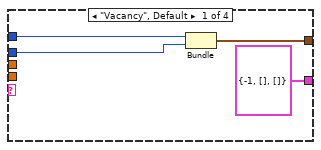
[diagram p13: hidden frame]
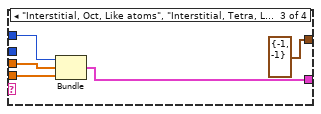
[diagram p14: hidden frame]
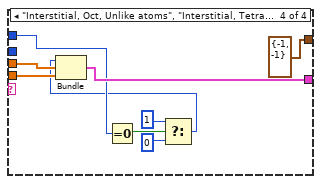
[diagram p15: hidden frame]
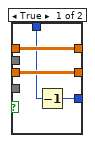
[diagram p18: hidden frame]
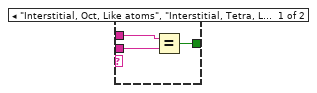
[diagram p19: hidden frame]
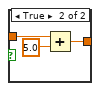
[diagram p20: hidden frame]
diagram:
  w31 = "Substitutional"
  w32 = "Vacancy"
  n1 = Unbundle By Name("Input Structure") -> ("Atoms Array"=w58:T4)
  n2 = Unbundle By Name("Input Structure") -> ("Atoms Array"=w57:T4, "# of atoms"=w56:i32)
  n3 = Unbundle By Name("Defect 1") -> ("Species"=w61:string, "Defect Type"=w7:string)
  n4 = Equal?(x=w7, y=w32) -> (x = y?=w35:bool)
  n5 = Equal?(x=w7, y=w31) -> (x = y?=w34:bool)
  n6 = Or(x=w35, y=w34) -> (x .or. y?=w12:bool)
  n7 = Not(x=w12) -> (.not. x?=w11:bool)
  n8 = for {
    tunnel: w58 -> [w62] mode=indexing
    tunnel: w61 -> [w64]
    tunnel: [w67] -> w9
    tunnel: [w66] -> _
    tunnel: [w63] -> _
    tunnel: w7 -> [w65]
    tunnel: [w62] -> w16
    i -> [w67]
    stop <- w66 stop-if-true
    n9 = Unbundle By Name(w62) -> ("Atom Name"=w63:string)
    n10 = case shown="\"Interstitial\", \"Interstitial, Oct, Unlike atoms\", \"Interstitial, Tetra, Unlike atoms\", \"Substitutional\"" w65 {
      tunnel: w63 -> [w69 w73]
      tunnel: [w68 w72] -> w66
      tunnel: w64 -> [w70 w71]
      frame "Interstitial, Oct, Like atoms", "Interstitial, Tetra, Like atoms", "Vacancy", Default {
        n11 = Equal?(x=w70, y=w69) -> (x = y?=w68:bool)
      }
      frame "Interstitial", "Interstitial, Oct, Unlike atoms", "Interstitial, Tetra, Unlike atoms", "Substitutional" {
        n12 = Not Equal?(x=w71, y=w73) -> (x != y?=w72:bool)
      }
    }
  }
  n13 = Unbundle By Name("Input Structure") -> ("Atoms Array"=w41:T4)
  n14 = Index Array(array=w41, index=w9) -> (element=w42:T5)
  n15 = Unbundle By Name(w16) -> ("Positions (Cartesian)"=w15:dbl[][])
  n16 = Unbundle By Name("Defect 2") -> ("Species"=w60:string, "Defect Type"=w33:string)
  n17 = Equal?(x=w33, y=w32) -> (x = y?=w29:bool)
  n18 = Equal?(x=w33, y=w31) -> (x = y?=w30:bool)
  n19 = Or(x=w29, y=w30) -> (x .or. y?=w21:bool)
  n20 = Not(x=w21) -> (.not. x?=w10:bool)
  n21 = And(x=w12, y=w21) -> (x .and. y?=w28:bool)
  n22 = Not(x=w28) -> (.not. x?=w27:bool)
  n23 = case shown="False" w27 {
    tunnel: "Input Structure" -> [_ w88]
    tunnel: [_ w76] -> w17
    frame False {
    }
    frame True {
      (unwired) -0.01 ("norm")
      n24 = Unbundle By Name(w88) -> ("Lattice vector a"=w87:dbl[], "Lattice vector b"=w86:dbl[], "Lattice vector c"=w85:dbl[])
      n25 = call-poly <vilib>:"Vector Norm.vi"("Input Vector"=w87) -> ("norm"=w84:dbl)  [unwired: 9 in, 1 out]
      n26 = call-poly <vilib>:"Vector Norm.vi"("Input Vector"=w86) -> ("norm"=w82:dbl)  [unwired: 9 in, 1 out]
      n27 = call-poly <vilib>:"Vector Norm.vi"("Input Vector"=w85) -> ("norm"=w79:dbl)  [unwired: 9 in, 1 out]
      n28 = Negate(x="Distance to check") -> (-x=w80:dbl)
      n29 = Add(x=w84, y="Distance to check") -> (x+y=w83:dbl)
      n30 = Add(x=w79, y="Distance to check") -> (x+y=w78:dbl)
      n31 = Add(x=w82, y="Distance to check") -> (x+y=w81:dbl)
      n32 = Bundle(w80, w83, w80, w81, w80, w78) -> (w75:cluster{dbl, dbl, dbl, dbl, dbl, dbl})  [unwired: 1 in]
      n33 = call "Supercell Structure into a Box.vi"("Keep old lattice vectors?"=TRUE, "Draw Box"=w75, "Subcrystal"=w88) -> ("Expanded cubic Structure"=w76:T1)  [unwired: 6 in, 2 out]
    }
  }
  n34 = Build Array(w7, w33) -> ()  [unwired: 1 out]
  n35 = Unbundle By Name(w17) -> ("Atoms Array"=w38:T4)
  n36 = case shown="\"Interstitial, Tetra, Like atoms\", \"Interstitial, Tetra, Unlike atoms\"" w7 {
    tunnel: w42 -> [w94 w112 w129]
    tunnel: [w92 w104 w118] -> w6
    tunnel: "Defect 1 Atom Index" -> [w90 w111 w128]
    tunnel: [w89 w100 w117] -> w5
    tunnel: "Input Structure" -> [_ w108 w119]
    tunnel: w17 -> [_ w96 w113]
    tunnel: w9 -> [_ w95 _]
    frame "Substitutional", "Vacancy", Default {
      n37 = Unbundle By Name(w94) -> ("Positions (Direct)"=w91:dbl[][], "Positions (Cartesian)"=w93:dbl[][])
      n38 = Index Array(array=w91, index (row)=w90) -> (element=w89:dbl[])  [unwired: 1 in]
      n39 = Index Array(array=w93, index (row)=w90) -> (element=w92:dbl[])  [unwired: 1 in]
    }
    frame "Interstitial, Oct, Like atoms", "Interstitial, Oct, Unlike atoms" {
      n40 = Unbundle By Name(w112) -> ("Positions (Cartesian)"=w110:dbl[][])
      n41 = Index Array(array=w110, index (row)=w111) -> (element=w99:dbl[])  [unwired: 1 in]
      n42 = Add(x=w99, y=dbl[] [0.001, 0.001, 0.001]) -> (x+y=w97:dbl[])
      n43 = call "Find interstitial position.vi"("Sublattice Index"=w95, "Interstitial Type"=T6."Octahedral (6 atoms)", "Suggested Location"=w97, "Input Structure"=w96) -> ("Actual Position"=w104:dbl[])  [unwired: 7 in]
      n44 = Unbundle By Name(w108) -> ("Lattice vector a"=w107:dbl[], "Lattice vector b"=w106:dbl[], "Lattice vector c"=w105:dbl[])
      n45 = Build Array(w104) -> (w103:dbl[][])
      n46 = call "Convert Cartesian to Direct.vi"("Lattice vector c"=w105, "Lattice vector b"=w106, "Lattice vector a"=w107, "Positions (Cartesian)"=w103) -> ("Positions (Direct)"=w102:dbl[][])  [unwired: 7 in]
      n47 = Index Array(array=w102, index (row)=0) -> (element=w100:dbl[])  [unwired: 1 in]
    }
    frame "Interstitial, Tetra, Like atoms", "Interstitial, Tetra, Unlike atoms" {
      n48 = Unbundle By Name(w129) -> ("Positions (Cartesian)"=w127:dbl[][])
      n49 = Index Array(array=w127, index (row)=w128) -> (element=w115:dbl[])  [unwired: 1 in]
      n50 = Add(x=w115, y=dbl[] [0.001, 0.001, 0.001]) -> (x+y=w114:dbl[])
      n51 = call "Find interstitial position.vi"("Interstitial Type"=T6."Tetrahedral (4 atoms)", "Suggested Location"=w114, "Input Structure"=w113) -> ("Actual Position"=w118:dbl[])  [unwired: 8 in]
      n52 = Unbundle By Name(w119) -> ("Lattice vector a"=w125:dbl[], "Lattice vector b"=w124:dbl[], "Lattice vector c"=w123:dbl[])
      n53 = Build Array(w118) -> (w122:dbl[][])
      n54 = call "Convert Cartesian to Direct.vi"("Lattice vector c"=w123, "Lattice vector b"=w124, "Lattice vector a"=w125, "Positions (Cartesian)"=w122) -> ("Positions (Direct)"=w121:dbl[][])  [unwired: 7 in]
      n55 = Index Array(array=w121, index (row)=0) -> (element=w117:dbl[])  [unwired: 1 in]
    }
  }
  "Defect 1 (Cart)" <- w6
  n56 = for {
    tunnel: w58 -> [w134] mode=indexing
    tunnel: w60 -> [w132]
    tunnel: [w135] -> w37
    tunnel: [w130] -> _
    tunnel: [w134] -> w59
    tunnel: [w131] -> _
    tunnel: w33 -> [w133]
    i -> [w135]
    stop <- w130 stop-if-true
    n57 = Unbundle By Name(w134) -> ("Atom Name"=w131:string)
    n58 = case shown="\"Interstitial\", \"Interstitial, Oct, Unlike atoms\", \"Interstitial, Tetra, Unlike atoms\", \"Substitutional\"" w133 {
      tunnel: w131 -> [w137 w141]
      tunnel: [w136 w140] -> w130
      tunnel: w132 -> [w138 w139]
      frame "Interstitial, Oct, Like atoms", "Interstitial, Tetra, Like atoms", "Vacancy", Default {
        n59 = Equal?(x=w138, y=w137) -> (x = y?=w136:bool)
      }
      frame "Interstitial", "Interstitial, Oct, Unlike atoms", "Interstitial, Tetra, Unlike atoms", "Substitutional" {
        n60 = Not Equal?(x=w139, y=w141) -> (x != y?=w140:bool)
      }
    }
  }
  "Numeric" <- w37
  n61 = Index Array(array=w38, index=w37) -> (element=w36:T5)
  n62 = case shown="True" w11 {
    tunnel: w6 -> [_ w143]
    tunnel: w15 -> [_ w142]
    frame False {
    }
    frame True {
      n63 = for {
        tunnel: w143 -> [w148]
        tunnel: w142 -> [w149] mode=indexing
        stop <- w144 stop-if-true
        n64 = Empty Array?(array=w148) -> (empty?=w147:bool)
        n65 = Equal?(x=w148, y=w149) -> (x = y?=w150:bool[])
        n66 = Not(x=w147) -> (.not. x?=w146:bool)
        n67 = And Array Elements(Boolean array=w150) -> (logical AND=w145:bool)
        n68 = And(x=w145, y=w146) -> (x .and. y?=w144:bool)
        n69 = case shown="True" w144 {
          frame False {
          }
          frame True {
            n70 = One Button Dialog(message="wtf") -> (true=w151:bool)  [unwired: 1 in]
            n71 = Stop(stop? (T)=w151) -> ()
          }
        }
      }
    }
  }
  n72 = Unbundle By Name(w36) -> ("Positions (Direct)"=w23:dbl[][], "Positions (Cartesian)"=w22:dbl[][])
  n73 = Unbundle By Name(w59) -> ("Positions (Direct)"=w25:dbl[][], "Positions (Cartesian)"=w13:dbl[][])
  n74 = case shown="False" w10 {
    tunnel: [w154 w155] -> w26
    tunnel: w13 -> [w154 _]
    tunnel: [w153 w156] -> w24
    tunnel: w25 -> [w153 _]
    tunnel: w23 -> [_ w156]
    tunnel: w22 -> [_ w155]
    frame False {
    }
    frame True {
    }
  }
  n75 = for {
    tunnel: w26 -> [w168] mode=indexing
    tunnel: w6 -> [w173]
    shift-right: [w166] -> w45
    shift-left: T3 [] -> [w165]
    tunnel: w24 -> [w163] mode=indexing
    tunnel: w10 -> [w160]
    tunnel: [w157] -> w20 mode=indexing
    i -> [w164]
    n76 = Subtract(x=w173, y=w168) -> (x-y=w172:dbl[])
    n77 = call-poly <vilib>:"Vector Norm.vi"("Input Vector"=w172) -> ("norm"=w157:dbl)  [unwired: 9 in, 1 out]
    n78 = Bundle("norm"=w157, w164, "Positions (Direct)"=w163, "Positions (Cartesian)"=w168) -> (w167:T7)  [unwired: 1 in]
    n79 = case shown="False" w160 {
      tunnel: "Minimum Distance" -> [w178 w181]
      tunnel: [w178 w180] -> w161
      frame False {
      }
      frame True {
        n80 = Subtract(x=w181, y=5.0) -> (x-y=w180:dbl)
      }
    }
    n81 = case shown="False" w160 {
      tunnel: [w174 w175] -> w158
      tunnel: "Maximum Distnce" -> [w174 w177]
      frame False {
      }
      frame True {
        n82 = Add(x=w177, y=5.0) -> (x+y=w175:dbl)
      }
    }
    n83 = Greater?(x=w157, y=w161) -> (0:w171:bool)
    n84 = Less?(x=w157, y=w158) -> (x < y?=w170:bool)
    n85 = And(x=w171, y=w170) -> (x .and. y?=w169:bool)
    n86 = case shown="True" w169 {
      tunnel: w167 -> [_ w185]
      tunnel: [w182 w184] -> w166
      tunnel: w165 -> [w182 w183]
      frame False {
      }
      frame True {
        n87 = Build Array (concatenate)(w183, w185) -> (w184:T3)
      }
    }
  }
  n88 = case shown="\"Vacancy\", Default" w7 {
    tunnel: w9 -> [w189 w197 w203 w208]
    tunnel: "Defect 1 Atom Index" -> [w188 w199 _ _]
    tunnel: [w187 w198 cluster{i32, "Defect 1 Atom Index":i32} {-1, "Defect 1 Atom Index"=-1} cluster{i32, "Defect 1 Atom Index":i32} {-1, "Defect 1 Atom Index"=-1}] -> w4
    tunnel: w5 -> [_ w191 w201 w206]
    tunnel: [T8 {-1, "Positions (Direct)"=[], "Positions (Cartesian)"=[]} w192 w204 w212] -> w3
    tunnel: w6 -> [_ w190 w200 w205]
    frame "Vacancy", Default {
      n89 = Bundle(w189, "Defect 1 Atom Index"=w188) -> (w187:cluster{i32, "Defect 1 Atom Index":i32})  [unwired: 1 in]
    }
    frame "Substitutional" {
      # "Atoms to add"
      # "Atoms to remove"
      n90 = Equal To 0?(x=w197) -> (x = 0?=w196:bool)
      n91 = Bundle(w197, "Defect 1 Atom Index"=w199) -> (w198:cluster{i32, "Defect 1 Atom Index":i32})  [unwired: 1 in]
      n92 = Select(t=1, s=w196, f=0) -> (s? t:f=w193:i32)
      n93 = Bundle(w193, "Positions (Direct)"=w191, "Actual Position"=w190) -> (w192:T9)  [unwired: 1 in]
    }
    frame "Interstitial, Oct, Like atoms", "Interstitial, Tetra, Like atoms" {
      n94 = Bundle(w203, "Positions (Direct)"=w201, "Actual Position"=w200) -> (w204:T9)  [unwired: 1 in]
    }
    frame "Interstitial, Oct, Unlike atoms", "Interstitial, Tetra, Unlike atoms" {
      n95 = Equal To 0?(x=w208) -> (x = 0?=w211:bool)
      n96 = Select(t=1, s=w211, f=0) -> (s? t:f=w207:i32)
      n97 = Bundle(w207, "Positions (Direct)"=w206, "Actual Position"=w205) -> (w212:T9)  [unwired: 1 in]
    }
  }
  n98 = Sort 1D Array(array=w20) -> (sorted array=→"Array":dbl[])
  n99 = Sort 1D Array(array=w45) -> (sorted array=w44:T3)
  "Defect Options" <- w44
  n100 = case shown="Default" w33 {
    selector: w33 -> [_ w219]
    tunnel: w44 -> [w216 w234]
    tunnel: [w217 w220] -> w43
    tunnel: w17 -> [_ w233]
    tunnel: w6 -> [_ w232]
    tunnel: "Input Structure" -> [_ w225]
    tunnel: [w214 w218] -> w18
    frame "Substitutional", "Vacancy" {
      # "Should just take the first smallest one"
      n101 = Empty Array?(array=w216) -> (empty?=w215:bool)
      n102 = Not(x=w215) -> (.not. x?=w214:bool)
      n103 = Index Array(array=w216) -> (element=w217:T7)  [unwired: 1 in]
    }
    frame Default {
      # "Need to check size."
      n104 = for {
        tunnel: w234 -> [w251] mode=indexing
        tunnel: w233 -> [w244]
        tunnel: [w237] -> w222
        tunnel: w232 -> [w243]
        tunnel: [w240] -> w224
        tunnel: [w235] -> w223
        tunnel: w219 -> [w239]
        tunnel: [w238] -> w218
        stop <- w238 stop-if-true
        n105 = case shown="\"Interstitial, Tetra, Like atoms\", \"Interstitial, Tetra, Unlike atoms\", Default" w239 {
          tunnel: [T6."Octahedral (6 atoms)" ("Interstitial Type") T6."Tetrahedral (4 atoms)" ("Interstitial Type")] -> w250
          frame "Interstitial, Oct, Like atoms", "Interstitial, Oct, Unlike atoms" {
          }
          frame "Interstitial, Tetra, Like atoms", "Interstitial, Tetra, Unlike atoms", Default {
          }
        }
        n106 = Unbundle(w251) -> (w240:i32, "Positions (Cartesian)"=w245:dbl[])  [unwired: 2 out]
        n107 = Add(x=w245, y=dbl[] [0.001, 0.001, 0.001]) -> (x+y=w249:dbl[])
        n108 = call "Find interstitial position.vi"("Interstitial Type"=w250, "Suggested Location"=w249, "Input Structure"=w244) -> ("Actual Position"=w237:dbl[])  [unwired: 8 in]
        n109 = local read "Minimum Distance"() -> (w242:dbl)
        n110 = local read "Maximum Distnce"() -> (w241:dbl)
        n111 = Subtract(x=w243, y=w237) -> (x-y=w236:dbl[])
        n112 = call-poly <vilib>:"Vector Norm.vi"("Input Vector"=w236) -> ("norm"=w235:dbl)  [unwired: 9 in, 1 out]
        n113 = Greater?(x=w235, y=w242) -> (0:w246:bool)
        n114 = Less?(x=w235, y=w241) -> (x < y?=w247:bool)
        n115 = And(x=w246, y=w247) -> (x .and. y?=w238:bool)
      }
      n116 = Unbundle By Name(w225) -> ("Lattice vector a"=w226:dbl[], "Lattice vector b"=w227:dbl[], "Lattice vector c"=w228:dbl[])
      n117 = Build Array(w222) -> (w229:dbl[][])
      n118 = call "Convert Cartesian to Direct.vi"("Lattice vector c"=w228, "Lattice vector b"=w227, "Lattice vector a"=w226, "Positions (Cartesian)"=w229) -> ("Positions (Direct)"=w230:dbl[][])  [unwired: 7 in]
      n119 = Index Array(array=w230, index (row)=0) -> (element=w221:dbl[])  [unwired: 1 in]
      n120 = Bundle("norm"=w223, w224, "Positions (Direct)"=w221, "Actual Position"=w222) -> (w220:T10)  [unwired: 1 in]
    }
  }
  "MATCH FOUND?!" <- w18
  n121 = Unbundle(w43) -> (w46:i32, "Positions (Direct)"=w47:dbl[], "Actual Position"=w14:dbl[])  [unwired: 1 out]
  "Defect 2 (Cart)" <- w14
  n122 = Subtract(x=w6, y=w14) -> (x-y=w50:dbl[])
  n123 = case shown="\"Substitutional\"" w33 {
    tunnel: w37 -> [w257 w265 w271 w274]
    tunnel: w46 -> [w256 w267 _ _]
    tunnel: [w255 w266 cluster{i32, "Defect 1 Atom Index":i32} {-1, "Defect 1 Atom Index"=-1} cluster{i32, "Defect 1 Atom Index":i32} {-1, "Defect 1 Atom Index"=-1}] -> w52
    tunnel: w14 -> [_ w258 w268 w279]
    tunnel: [T8 {-1, "Positions (Direct)"=[], "Positions (Cartesian)"=[]} w260 w272 w278] -> w51
    tunnel: w47 -> [_ w259 w269 w280]
    frame "Vacancy", Default {
      n124 = Bundle(w257, w256) -> (w255:cluster{i32, i32})  [unwired: 1 in]
    }
    frame "Substitutional" {
      # "Atoms to add"
      # "Atoms to remove"
      n125 = Equal To 0?(x=w265) -> (x = 0?=w264:bool)
      n126 = Bundle(w265, w267) -> (w266:cluster{i32, i32})  [unwired: 1 in]
      n127 = Select(t=1, s=w264, f=0) -> (s? t:f=w261:i32)
      n128 = Bundle(w261, "Positions (Direct)"=w259, "Actual Position"=w258) -> (w260:T9)  [unwired: 1 in]
    }
    frame "Interstitial, Oct, Like atoms", "Interstitial, Tetra, Like atoms" {
      n129 = Bundle(w271, "Positions (Direct)"=w269, "Actual Position"=w268) -> (w272:T9)  [unwired: 1 in]
    }
    frame "Interstitial, Oct, Unlike atoms", "Interstitial, Tetra, Unlike atoms" {
      n130 = Equal To 0?(x=w274) -> (x = 0?=w277:bool)
      n131 = Select(t=1, s=w277, f=0) -> (s? t:f=w273:i32)
      n132 = Bundle(w273, "Positions (Direct)"=w280, "Actual Position"=w279) -> (w278:T9)  [unwired: 1 in]
    }
  }
  n133 = call-poly <vilib>:"Vector Norm.vi"("Input Vector"=w50) -> ("norm"=→"Distance between defects (A)":dbl)  [unwired: 9 in, 1 out]
  n134 = case shown="True" w10 {
    tunnel: w14 -> [_ w283]
    tunnel: w13 -> [_ w282]
    frame False {
    }
    frame True {
      n135 = for {
        tunnel: w283 -> [w288]
        tunnel: w282 -> [w289] mode=indexing
        stop <- w284 stop-if-true
        n136 = Empty Array?(array=w288) -> (empty?=w287:bool)
        n137 = Equal?(x=w288, y=w289) -> (x = y?=w290:bool[])
        n138 = Not(x=w287) -> (.not. x?=w286:bool)
        n139 = And Array Elements(Boolean array=w290) -> (logical AND=w285:bool)
        n140 = And(x=w285, y=w286) -> (x .and. y?=w284:bool)
        n141 = case shown="True" w284 {
          frame False {
          }
          frame True {
            n142 = One Button Dialog(message="wtf") -> (true=w291:bool)  [unwired: 1 in]
            n143 = Stop(stop? (T)=w291) -> ()
          }
        }
      }
    }
  }
  n144 = for {
    tunnel: w57 -> [w324] mode=indexing
    tunnel: [w322] -> w54 mode=indexing
    tunnel: w4 -> [w321]
    tunnel: w52 -> [w320]
    tunnel: w3 -> [w313]
    tunnel: w51 -> [w312]
    shift-right: [w302] -> w55
    shift-left: w56 -> [w294]
    i -> [w307]
    w325 = dbl[][] []
    # "Remove atoms which match the atom and species indicies"
    n145 = Unbundle(w321) -> (w319:i32, "Defect 1 Atom Index"=w315:i32)
    n146 = Unbundle(w320) -> (w318:i32, "Defect 1 Atom Index"=w314:i32)
    n147 = Unbundle(w313) -> (w311:i32, "Positions (Direct)"=w309:dbl[], "Actual Position"=w299:dbl[])
    n148 = Unbundle(w312) -> (w306:i32, "Positions (Direct)"=w304:dbl[], "Actual Position"=w297:dbl[])
    n149 = Unbundle By Name(w324) -> ("Atom Name"=w323:string, "Positions (Direct)"=w327:dbl[][], "Positions (Cartesian)"=w326:dbl[][])
    n150 = Equal?(x=w319, y=w307) -> (x = y?=w317:bool)
    n151 = Equal?(x=w318, y=w307) -> (x = y?=w316:bool)
    n152 = Equal?(x=w307, y=w311) -> (x = y?=w310:bool)
    n153 = Equal?(x=w307, y=w306) -> (x = y?=w305:bool)
    n154 = for {
      tunnel: w327 -> [w367] mode=indexing
      tunnel: w326 -> [w364] mode=indexing
      shift-right: [w363] -> w300
      shift-left: w325 -> [w362]
      shift-right: [w366] -> w301
      shift-left: w325 -> [w365]
      tunnel: w317 -> [w360]
      tunnel: w316 -> [w359]
      tunnel: w315 -> [w356]
      tunnel: w314 -> [w354]
      shift-right: [w350] -> w293
      shift-left: w294 -> [w351]
      i -> [w353]
      n155 = Equal?(x=w356, y=w353) -> (x = y?=w355:bool)
      n156 = Equal?(x=w354, y=w353) -> (x = y?=w352:bool)
      n157 = And(x=w360, y=w355) -> (x .and. y?=w358:bool)
      n158 = And(x=w359, y=w352) -> (x .and. y?=w357:bool)
      n159 = Or(x=w358, y=w357) -> (x .or. y?=w361:bool)
      n160 = case shown="False" w361 {
        tunnel: w367 -> [_ w378]
        tunnel: [w371 w377] -> w366
        tunnel: w365 -> [w371 w376]
        tunnel: w364 -> [_ w375]
        tunnel: [w370 w374] -> w363
        tunnel: w362 -> [w370 w373]
        tunnel: w351 -> [w369 w372]
        tunnel: [w368 w372] -> w350
        frame True {
          n161 = Decrement(x=w369) -> (x-1=w368:i32)
        }
        frame False {
          n162 = Build Array (concatenate)(w376, w378) -> (w377:dbl[][])
          n163 = Build Array (concatenate)(w373, w375) -> (w374:dbl[][])
        }
      }
    }
    n164 = case shown="True" w310 {
      tunnel: w301 -> [w341 w349]
      tunnel: w309 -> [_ w348]
      tunnel: [w341 w347] -> w308
      tunnel: w293 -> [w340 w346]
      tunnel: [w340 w345] -> w303
      tunnel: w300 -> [w339 w344]
      tunnel: w299 -> [_ w343]
      tunnel: [w339 w342] -> w298
      frame False {
      }
      frame True {
        n165 = Increment(x=w346) -> (x+1=w345:i32)
        n166 = Build Array (concatenate)(w349, w348) -> (w347:dbl[][])
        n167 = Build Array (concatenate)(w344, w343) -> (w342:dbl[][])
      }
    }
    n168 = case shown="True" w305 {
      tunnel: w308 -> [w330 w338]
      tunnel: w304 -> [_ w337]
      tunnel: [w330 w336] -> w296
      tunnel: w303 -> [w329 w335]
      tunnel: [w329 w334] -> w302
      tunnel: w298 -> [w328 w333]
      tunnel: w297 -> [_ w332]
      tunnel: [w328 w331] -> w295
      frame False {
      }
      frame True {
        n169 = Increment(x=w335) -> (x+1=w334:i32)
        n170 = Build Array (concatenate)(w338, w337) -> (w336:dbl[][])
        n171 = Build Array (concatenate)(w333, w332) -> (w331:dbl[][])
      }
    }
    n172 = Bundle(cluster=w324, "Atom Name"=w323, "Positions (Direct)"=w296, "Positions (Cartesian)"=w295) -> (w322:T5)
  }
  n173 = Bundle By Name(cluster="Input Structure", "Atoms Array"=w54, "# of atoms"=w55) -> (w2:T1)
  n174 = call "Map Structure to [0,1).vi"("Structure"=w2) -> ("Structure mapped to [0,1)"=→"Defectuous Structure":T11)  [unwired: 10 in]
